vi "陀螺仪.vi"() -> ()   [LabVIEW 2017]
uses:
  <vilib>/myRIO/Instrument Drivers/Onboard IO/I2C/typedefs/I2C User Configuration.ctl
  <vilib>/myRIO/Instrument Drivers/Onboard IO/I2C/typedefs/I2C Transfer Rate.ctl
  <vilib>/Platform/TimedLoop/XDataNode/timing_clust.ctl
  <vilib>/Platform/TimedLoop/XDataNode/nitl_modes.ctl
  <vilib>/Platform/TimedLoop/XDataNode/wakeup.ctl
  <vilib>/myRIO/Instrument Drivers/Onboard IO/I2C/typedefs/I2C Reference.ctl
  <vilib>/myRIO/Common/Instrument Driver Framework/Utilities/typedefs/myRIO Generic Hardware Reference.ctl
  <vilib>/myRIO/Common/Instrument Driver Framework/Utilities/typedefs/Hardware Version Enum.ctl
  <vilib>/myRIO/Common/Instrument Driver Framework/Utilities/typedefs/myRIO v1.0 Reference.ctl
  <vilib>/myRIO/Common/Instrument Driver Framework/Utilities/typedefs/Generic FPGA Reference.ctl
  <vilib>/myRIO/Common/Instrument Driver Framework/myRIO v1.0/I2C/typedefs/I2C Channels Enum.ctl
  <vilib>/myRIO/Instrument Drivers/Onboard IO/I2C/typedefs/I2C Configuration.ctl
  <vilib>/userdefined/High Color/nirio_resource_hc.ctl
  <vilib>/myRIO/Common/Instrument Driver Framework/myRIO v1.0/I2C/vis/myRIO v1.1 Open I2C.vi
  <vilib>/myRIO/Common/Instrument Driver Framework/Utilities/vis/Validate Channels.vi
  <vilib>/myRIO/Common/Instrument Driver Framework/myRIO v1.0/I2C/vis/myRIO v1.0 Reserve I2C.vi
  <vilib>/myRIO/Common/Instrument Driver Framework/myRIO v1.0/UART/vis/myRIO v1.0 Close UART.vi
  <vilib>/myRIO/Common/Instrument Driver Framework/myRIO v1.0/I2C/vis/myRIO v1.0 Build MUX Configuration I2C.vi
  <vilib>/myRIO/Common/Instrument Driver Framework/myRIO v1.0/Resource Manager/vis/myRIO v1.0 Reserve Channel List.vi
  <vilib>/myRIO/Common/Instrument Driver Framework/myRIO v1.0/Resource Manager/vis/myRIO v1.0 Create Configuration List.vi
  <vilib>/myRIO/Common/Instrument Driver Framework/myRIO v1.0/Resource Manager/vis/myRIO v1.0 Reserve Channel.vi
  <vilib>/myRIO/Common/Instrument Driver Framework/myRIO v1.0/Resource Manager/vis/myRIO v1.0 Unreserve Channel.vi
  <vilib>/myRIO/Common/Instrument Driver Framework/myRIO v1.0/Resource Manager/vis/myRIO v1.0 Build Mutex Name.vi
  <vilib>/Utility/VariantDataType/GetNumericInfo.vi
  <vilib>/Utility/error.llb/Error Cluster From Error Code.vi
  <vilib>/myRIO/Common/Instrument Driver Framework/myRIO v1.0/myRIO v1.1 Open.vi
  <vilib>/myRIO/Common/Instrument Driver Framework/Utilities/vis/IO Manager.vi
  <vilib>/myRIO/Common/Instrument Driver Framework/Utilities/vis/Configuration Manager.vi
  <vilib>/myRIO/Common/Instrument Driver Framework/myRIO v1.0/Resource Manager/vis/myRIO v1.0 Configure IO.vi
  <vilib>/myRIO/Common/Instrument Driver Framework/myRIO v1.0/myRIO v1.0 Close.vi
  <vilib>/myRIO/Common/Instrument Driver Framework/myRIO v1.0/I2C/vis/myRIO v1.0 Configure I2C.vi
  <vilib>/myRIO/Common/Instrument Driver Framework/myRIO v1.0/I2C/vis/myRIO v1.0 Write I2C.vi
  <vilib>/myRIO/Common/Instrument Driver Framework/myRIO v1.0/I2C/vis/myRIO v1.0 Read I2C.vi
  <vilib>/myRIO/Common/Instrument Driver Framework/Utilities/vis/FPGA Ref Manager.vi
  <vilib>/myRIO/Common/Instrument Driver Framework/myRIO v1.0/myRIO v1.0 Reset FPGA.vi
  <vilib>/myRIO/Common/Instrument Driver Framework/myRIO v1.0/IRQ/vis/myRIO v1.0 IRQ Info FGV.vi
  <vilib>/myRIO/Common/Instrument Driver Framework/myRIO v1.0/IRQ/vis/myRIO v1.0 Timer IRQ Info FGV.vi
  <vilib>/myRIO/Common/Instrument Driver Framework/myRIO v1.0/IRQ/vis/myRIO v1.0 ISR Agent.vi
  <vilib>/Platform/TimedLoop/XDataNode/XDataNode.xnode
  <vilib>/myRIO/Instrument Drivers/Onboard IO/I2C/vis/myRIO I2C Open.xnode
  <vilib>/myRIO/Instrument Drivers/Onboard IO/I2C/I2C.lvlib
  <vilib>/ptbypt/NI_PtbyPt.lvlib
  <vilib>/Platform/TimedLoop/XDataNode/XDNodeRunTimeDep.lvlib
  <vilib>/rvi/interface/nirviOpenFPGA/nirviOpenFPGA.xnode
  <vilib>/FPGAPlugInAG/myRIO-1900/niLvFpga_Open_myRIO-1900.vi
  <vilib>/rvi/interface/common/dynamic/niFpgaDynamicAddResources.vi
  <vilib>/myRIO/Instrument Drivers/Utilities/Utilities.lvlib
  <vilib>/rvi/interface/nirviCloseFPGA/nirviCloseFPGA.xnode
  <vilib>/FPGAPlugInAG/Dynamic/niLvFpga_Close_Dynamic.vi
panel:
  in  "y":sgl=26.5
  in  "x":sgl=-16.0
  in  "initialize":bool caption="初始化"
  in  "停止":bool
  out "加速度":cluster{i16, i16, i16}(graph)
  out "角度":T1(graph)
  out "角速度":cluster{"x":dbl, sgl, sgl}(graph)
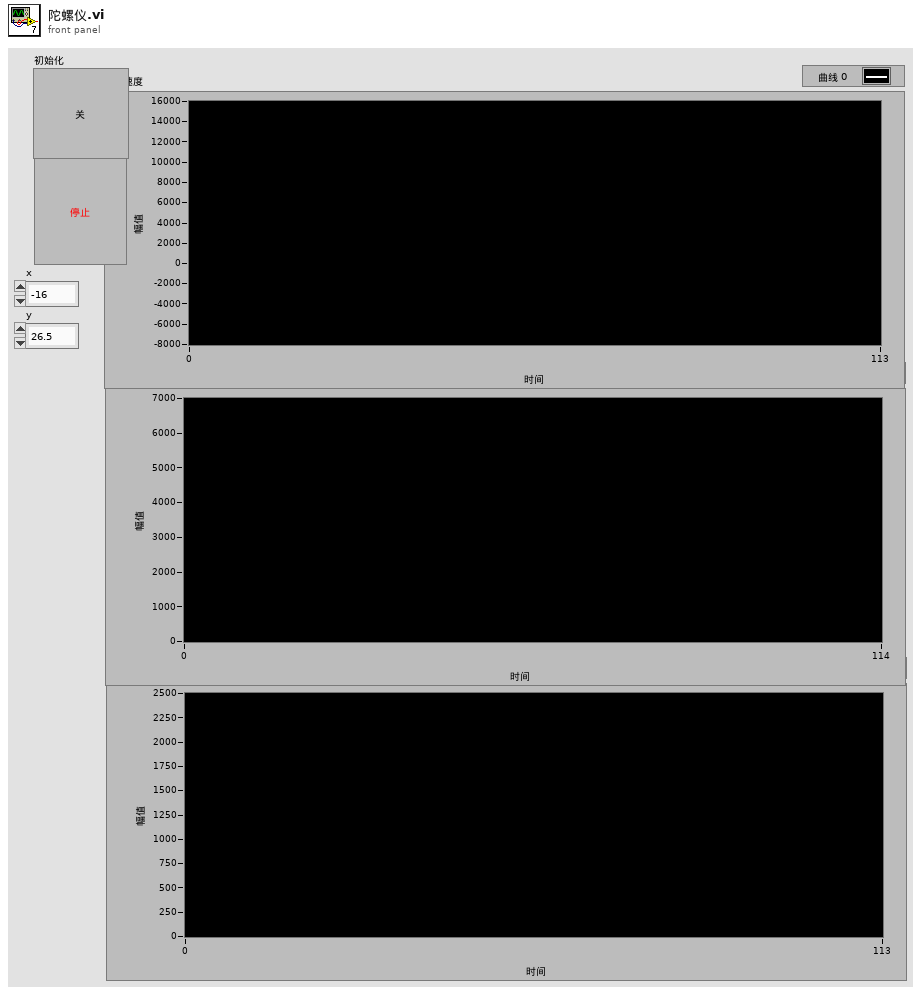
[diagram p1: front panel]
types:
  T1 = cluster{"integral x(t)":dbl, "integral x(t)":dbl, "integral x(t)":dbl}
  T2 = typedef "I2C.lvlib/I2C User Configuration.ctl" = cluster{"I2C Transfer Rate":T3}
  T3 = typedef "I2C.lvlib/I2C Transfer Rate.ctl" = enum16{"Standard mode (100 kbps)", "Fast mode (400 kbps)"}
  T4 = typedef "I2C.lvlib/I2C Reference.ctl" = cluster{"myRIO Reference":T5, "I2C Channels Enum":T9, "I2C Configuration":T10}
  T5 = typedef "myRIO Generic Hardware Reference.ctl" = cluster{"myRIO Model":T6, "myRIO Hardware Reference":T7}
  T6 = typedef "Hardware Version Enum.ctl" = enum16{"Unknown", "myRIO-1900", "myRIO-1950", "roboRIO", "NI ELVIS RIO CM"}
  T7 = typedef "myRIO v1.0 Reference.ctl" = cluster{"Generic FPGA Reference":T8, "Allow multiple opens":bool}
  T8 = typedef "Generic FPGA Reference.ctl" = refnum<k20>
  T9 = typedef "I2C Channels Enum.ctl" = enum16{"Not Connected", "A/I2C", "B/I2C", "I2C/I2C"}
  T10 = typedef "I2C.lvlib/I2C Configuration.ctl" = cluster{"I2C Transfer Rate":T3}
  T11 = typedef "XDNodeRunTimeDep.lvlib/timing_clust.ctl" = cluster{"Expected End [f-1]":u64, "Actual End [f-1]":u64, "Finished Late? [f-1]":bool, "Expected End [i-1]":u64, "Actual End [i-1]":u64, "Finished Late? [i-1]":bool, "Expected Start [i]":u64, "Actual Start [i]":u64, "Expected Start [f]":u64, "Actual Start [f]":u64, "Source Name":string, "Structure Name":string, "Period":i64, "Deadline":i64, "Offset":i64, "Start":i64, "Priority":i32, "Timeout":i32, "Mode":T12, "Wakeup Reason":T13, "Error":errorcluster, "Source Type":string, "Secondary Source Type":string, "Global End Time":u64, "Global Start Time":u64, "Frame Duration":u64, "Iteration Duration":u64, "Assigned CPU":i32, "I/O Scan Engine Mode":u32}
  T12 = typedef "XDNodeRunTimeDep.lvlib/nitl_modes.ctl" = enum32{"No Change", "Process missed periods, maintain original phase", "Discard missed periods, maintain original phase", "Process missed periods, ignore original phase", "Discard missed periods, ignore original phase"}
  T13 = typedef "XDNodeRunTimeDep.lvlib/wakeup.ctl" = enum32{"Normal", "Aborted", "Asynchronous wakeup", "Timing source error", "Timed loop error", "Timeout"}
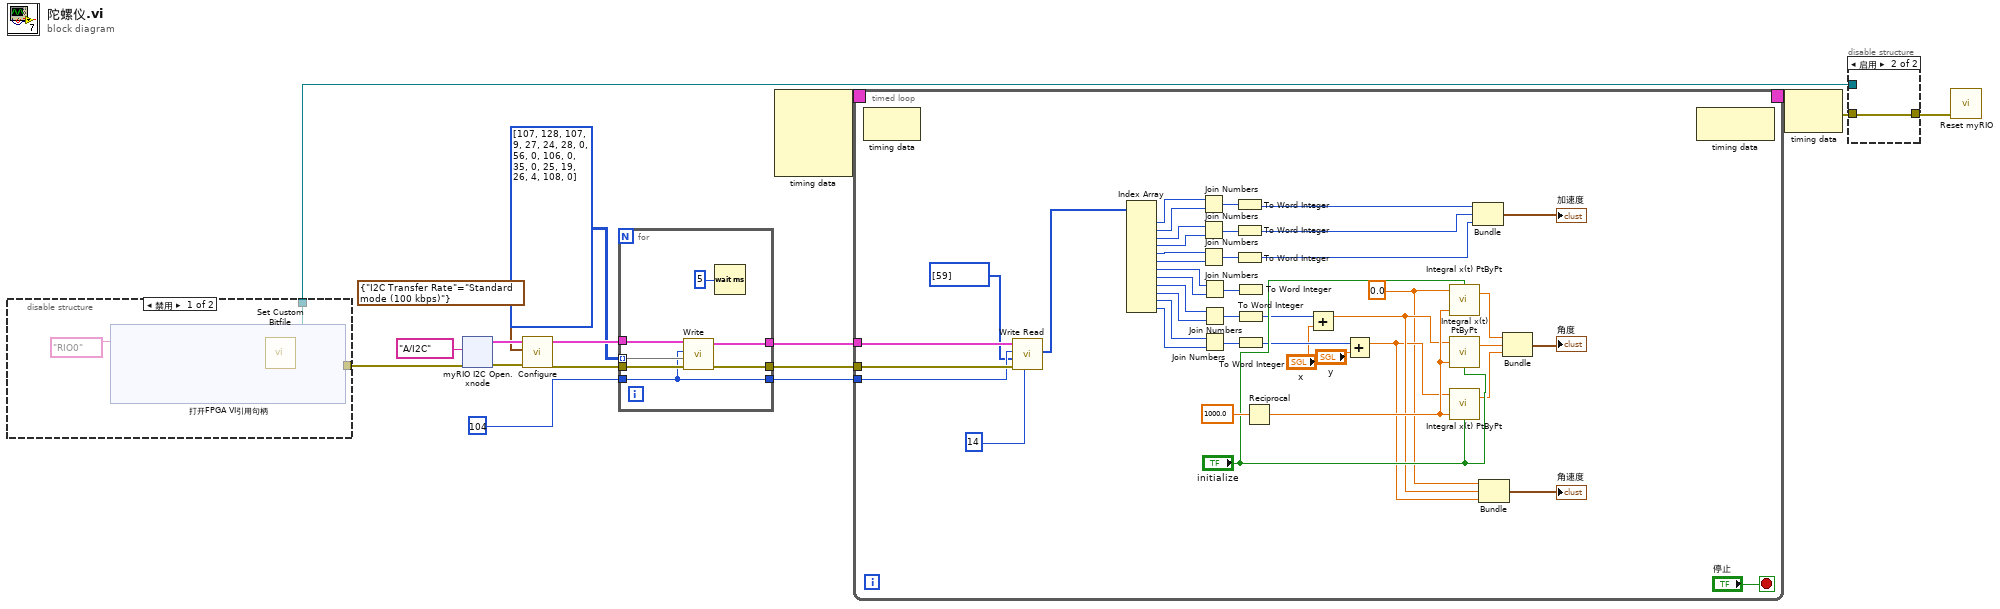
[diagram p0: block diagram]
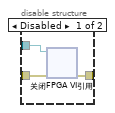
[diagram p2: hidden frame]
diagram:
  n1 = disable-structure shown="禁用" {
    disable-tunnel: [w20 _] -> w4
    disable-tunnel: [w18 _] -> w1
    frame Disabled {
      n2 = xnode "打开FPGA VI引用句柄"("资源名称"=tag "RIO0") -> ("FPGA VI引用输出"=w19:refnum<k20>, "错误输出"=w21:errorcluster)  [unwired: 1 in]
      n3 = call <vilib>:"Set Custom Bitfile.vi"("error in (no error)"=w21, "Custom FPGA Reference In"=w19) -> ("error out"=w20:errorcluster, "Custom FPGA Reference Out"=w18:refnum<k20>)  [unwired: 8 in]
    }
    frame Enabled {
    }
  }
  n4 = xnode "myRIO I2C Open.xnode"("error in (no error)"=w4, "Channel Name"=tag "A/I2C") -> ("error out"=w17:errorcluster, "I2C Ref Out"=w16:T4)  [unwired: 1 in]
  n5 = call <vilib>:"Configure.vi"("error in (no error)"=w17, "I2C User Configuration"=T2 {"I2C Transfer Rate"=enum."Standard mode (100 kbps)"}, "I2C Ref In"=w16) -> ("error out"=w12:errorcluster, "I2C Ref Out"=w13:T4)  [unwired: 7 in]
  n6 = for {
    tunnel: w13 -> [w29]
    tunnel: w12 -> [w28]
    tunnel: [w27] -> w11
    tunnel: [w26] -> w10
    tunnel: u8 104 ("Slave Address (7-bit)") -> [w23]
    tunnel: u8[][] [[107, 128], [107, 9], [27, 24], [28, 0], [56, 0], [106, 0], [35, 0], [25, 19], [26, 4], [108, 0]] ("Bytes to Write") -> [w24] mode=indexing
    tunnel: [w23] -> w7
    n7 = call <vilib>:"Write.vi"("error in (no error)"=w28, "Bytes to Write"=w24, "Slave Address (7-bit)"=w23, "I2C Ref In"=w29) -> ("error out"=w26:errorcluster, "I2C Ref Out"=w27:T4)  [unwired: 6 in]
    n8 = Wait (ms)(milliseconds to wait=u32 5 ("等待时间（毫秒）")) -> ()  [unwired: 1 out]
  }
  n9 = node-c288() -> (w6:T11)  [unwired: 4 in]
  n10 = timed-loop {
    timing: w6 -> [_]
    timing-out: [_] -> w5
    tunnel: w11 -> [w73]
    tunnel: w10 -> [w72]
    tunnel: w7 -> [w71]
    stop <- "停止" stop-if-true
    w30 = 0.0 ("x")
    n11 = node-c288() -> ()  [unwired: 1 in, 1 out]
    n12 = call <vilib>:"Write Read.vi"("Byte Count"=u32 14, "error in (no error)"=w72, "Bytes to Write"=u8[] [59], "Slave Address (7-bit)"=w71, "I2C Ref In"=w73) -> ("Bytes Read"=w69:u8[])  [unwired: 3 in, 2 out]
    n13 = Index Array(array=w69) -> (element #1=w68:u8, element #2=w67:u8, element #3=w66:u8, element #4=w65:u8, element #5=w64:u8, element #6=w63:u8, element #7=w62:u8, element #8=w61:u8, element #9=w60:u8, element #10=w59:u8, element #11=w58:u8, element #12=w57:u8)  [unwired: 12 in]
    n14 = Join Numbers(hi=w68, lo=w67) -> ((hi.lo)=w55:u16)
    n15 = Join Numbers(hi=w66, lo=w65) -> ((hi.lo)=w54:u16)
    n16 = Join Numbers(hi=w64, lo=w63) -> ((hi.lo)=w53:u16)
    n17 = Join Numbers(hi=w62, lo=w61) -> ((hi.lo)=w52:u16)
    n18 = Join Numbers(hi=w60, lo=w59) -> ((hi.lo)=w51:u16)
    n19 = Join Numbers(hi=w58, lo=w57) -> ((hi.lo)=w50:u16)
    n20 = To Word Integer(number=w55) -> (16bit integer=w49:i16)
    n21 = To Word Integer(number=w54) -> (16bit integer=w48:i16)
    n22 = To Word Integer(number=w53) -> (16bit integer=w47:i16)
    n23 = To Word Integer(number=w52) -> ()  [unwired: 1 out]
    n24 = To Word Integer(number=w51) -> (16bit integer=w36:i16)
    n25 = To Word Integer(number=w50) -> (16bit integer=w35:i16)
    n26 = Reciprocal(x=1000.0) -> (1/x=w45:dbl)
    n27 = Add(x=w36, y="y") -> (x+y=w34:sgl)
    n28 = Add(x=w35, y="x") -> (x+y=w32:sgl)
    n29 = call <vilib>:"Integral x(t) PtByPt.vi"("initialize"="initialize", "dt"=w45, "x"=w30) -> ("integral x(t)"=w43:dbl)  [unwired: 1 in, 1 out]
    n30 = call <vilib>:"Integral x(t) PtByPt.vi"("initialize"="initialize", "dt"=w45, "x"=w34) -> ("integral x(t)"=w42:dbl)  [unwired: 1 in, 1 out]
    n31 = call <vilib>:"Integral x(t) PtByPt.vi"("initialize"="initialize", "dt"=w45, "x"=w32) -> ("integral x(t)"=w37:dbl)  [unwired: 1 in, 1 out]
    n32 = Bundle(w49, w48, w47) -> (→"加速度":cluster{i16, i16, i16})  [unwired: 1 in]
    n33 = Bundle("x"=w30, w34, w32) -> (→"角速度":cluster{"x":dbl, sgl, sgl})  [unwired: 1 in]
    n34 = Bundle("integral x(t)"=w43, "integral x(t)"=w42, "integral x(t)"=w37) -> (→"角度":T1)  [unwired: 1 in]
    n35 = node-c288() -> ()  [unwired: 1 in, 1 out]
  }
  n36 = node-c288(w5) -> (w3:errorcluster)
  n37 = disable-structure shown="启用" {
    disable-tunnel: w3 -> [w78 w79]
    disable-tunnel: [w77 w79] -> w2
    disable-tunnel: w1 -> [w76 _]
    frame Disabled {
      n38 = xnode "关闭FPGA VI引用"("FPGA VI引用输入"=w76, "错误输入"=w78) -> ("错误输出"=w77:errorcluster)
    }
    frame Enabled {
    }
  }
  n39 = call <vilib>:"Reset myRIO.vi"("error in (no error)"=w2) -> ()  [unwired: 10 in, 1 out]
